vi "MP_SYNCHRONISED_TEST.vi"(5 "error in (no error)":errorcluster, 6 "TB: IP ADDRESS":string="192.168.0.100", 7 "Chopper Serial Number":string="26", 8 "Connection ID TB":refnum<k5>, 9 "Connection ID CC":refnum<k5>) -> (0 "PASS / FAIL":bool, 1 "error out":errorcluster, 2 "Connection ID CC 2":refnum<k5>, 3 "Connection ID TB 2":refnum<k5>, 4 "concatenated string":string)   [LabVIEW 2013]
panel:
  out "PROGRESS":i32(slide) scale=0.0..5.0
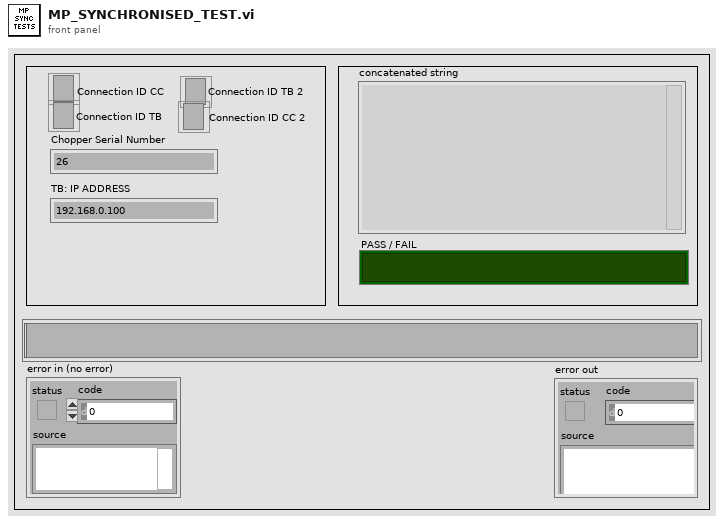
[diagram p1: front panel]
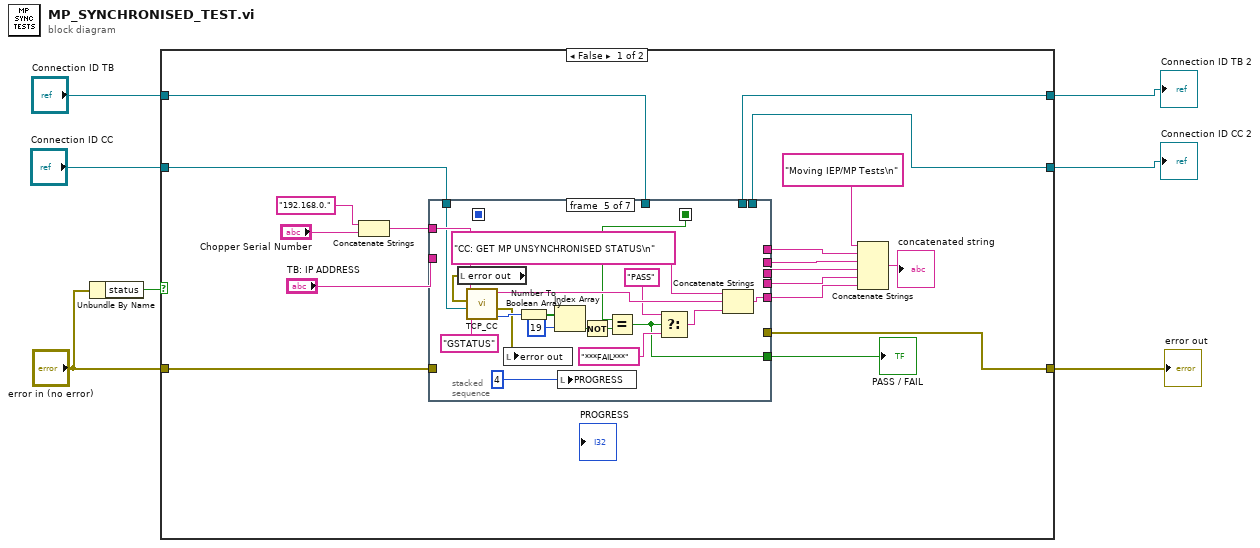
[diagram p0: block diagram]
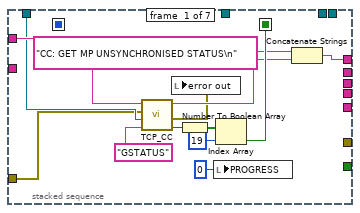
[diagram p2: hidden frame]
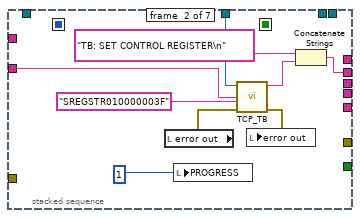
[diagram p3: hidden frame]
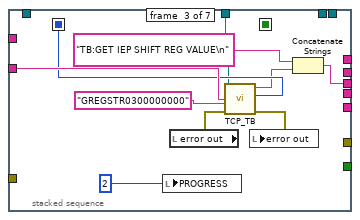
[diagram p4: hidden frame]
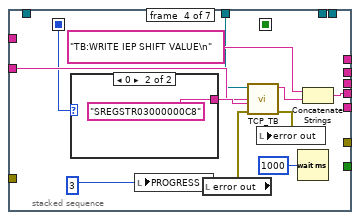
[diagram p5: hidden frame]
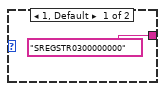
[diagram p6: hidden frame]
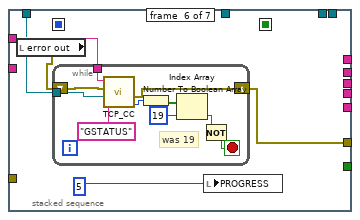
[diagram p7: hidden frame]
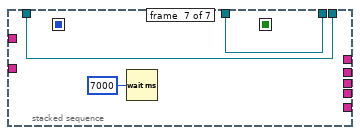
[diagram p8: hidden frame]
diagram:
  n1 = Unbundle By Name("error in (no error)") -> ("status"=w2:bool)
  n2 = case shown="False" w2 {
    tunnel: "Connection ID CC" -> [w13 w109]
    tunnel: "Connection ID TB" -> [w12 w110]
    tunnel: [w9 w110] -> w5
    tunnel: [w8 w109] -> w4
    tunnel: "error in (no error)" -> [w11 w108]
    tunnel: [w10 w108] -> w3
    frame False {
      n3 = Concatenate Strings("192.168.0.", "Chopper Serial Number") -> (w14:string)
      n4 = stacked-sequence {
        seq-local: [w33 _ _ _ _ _ _] -> [_ _ _ _ w79 _ _]
        seq-local: [_ _ w55 _ _ _ _] -> [_ _ _ w66 _ _ _]
        tunnel: "TB: IP ADDRESS" -> [_ w46 w56 w67 _ _ _]
        tunnel: w14 -> [w37 _ _ _ w88 w94 _]
        tunnel: [w30 _ _ _ _ _ _] -> w25
        tunnel: [_ w43 _ _ _ _ _] -> w24
        tunnel: [_ _ w52 _ _ _ _] -> w23
        tunnel: [_ _ _ w63 _ _ _] -> w22
        tunnel: [_ _ _ _ w82 _ _] -> w21
        tunnel: [_ _ _ _ w75 _ _] -> w16
        tunnel: w13 -> [w28 _ _ _ w73 w92 w105]
        tunnel: w12 -> [_ w41 w50 w60 _ _ w106]
        tunnel: w11 -> [w27 _ _ _ _ _ _]
        tunnel: [_ _ _ _ _ w91 _] -> w10
        tunnel: [_ _ _ _ _ _ w106] -> w9
        tunnel: [_ _ _ _ _ _ w105] -> w8
        frame #0 {
          n5 = call "TCP_CC.vi"("COMMAND"="GSTATUS", "connection ID"=w28, "error in (no error)"=w27, "IP ADDRESS"=w37) -> ("number"=w36:u32, "error out"=w26:errorcluster, "The Response:"=w31:string)  [unwired: 1 out]
          n6 = local write "error out"(w26) -> ()
          n7 = Number To Boolean Array(number=w36) -> (Boolean array=w35:bool[])
          n8 = local write "PROGRESS"(0 ("PROGRESS")) -> ()
          n9 = Index Array(array=w35, index=19) -> (element=w33:bool)
          n10 = Concatenate Strings("CC: GET MP UNSYNCHRONISED STATUS\n", w31) -> (w30:string)
        }
        frame #1 {
          n11 = local read "error out"() -> (w39:errorcluster)
          n12 = local write "PROGRESS"(1 ("PROGRESS")) -> ()
          n13 = call "TCP_TB.vi"("IP ADDRESS"=w46, "error in (no error)"=w39, "COMMAND"="SREGSTR010000003F", "Connection ID IN"=w41) -> ("error out"=w40:errorcluster, "Their Response:"=w44:string)  [unwired: 2 in, 1 out]
          n14 = local write "error out"(w40) -> ()
          n15 = Concatenate Strings("TB: SET CONTROL REGISTER\n" ("COMMAND"), w44) -> (w43:string)
        }
        frame #2 {
          n16 = local write "PROGRESS"(2 ("PROGRESS")) -> ()
          n17 = local read "error out"() -> (w48:errorcluster)
          n18 = call "TCP_TB.vi"("IP ADDRESS"=w56, "error in (no error)"=w48, "COMMAND"="GREGSTR0300000000", "Connection ID IN"=w50) -> ("error out"=w49:errorcluster, "Decimal Number"=w55:u32, "Their Response:"=w54:string)  [unwired: 2 in]
          n19 = local write "error out"(w49) -> ()
          n20 = Concatenate Strings("TB:GET IEP SHIFT REG VALUE\n" ("COMMAND"), w54) -> (w52:string)
        }
        frame #3 {
          n21 = case shown="0" w66 {
            tunnel: ["SREGSTR0300000000" ("COMMAND") "SREGSTR03000000C8" ("COMMAND")] -> w68
            frame 1, Default {
            }
            frame 0 {
            }
          }
          n22 = local write "PROGRESS"(3 ("PROGRESS")) -> ()
          n23 = local read "error out"() -> (w58:errorcluster)
          n24 = call "TCP_TB.vi"("IP ADDRESS"=w67, "error in (no error)"=w58, "COMMAND"=w68, "Connection ID IN"=w60) -> ("error out"=w59:errorcluster, "Their Response:"=w65:string)  [unwired: 2 in, 1 out]
          n25 = local write "error out"(w59) -> ()
          n26 = Wait (ms)(milliseconds to wait=u32 1000 ("millisecond multiple")) -> ()  [unwired: 1 out]
          n27 = Concatenate Strings("TB:WRITE IEP SHIFT VALUE\n", w65) -> (w63:string)
        }
        frame #4 {
          n28 = local read "error out"() -> (w71:errorcluster)
          n29 = call "TCP_CC.vi"("COMMAND"="GSTATUS", "connection ID"=w73, "error in (no error)"=w71, "IP ADDRESS"=w88) -> ("number"=w87:u32, "error out"=w72:errorcluster, "The Response:"=w83:string)  [unwired: 1 out]
          n30 = local write "error out"(w72) -> ()
          n31 = Number To Boolean Array(number=w87) -> (Boolean array=w86:bool[])
          n32 = Index Array(array=w86, index=19) -> (element=w81:bool)
          n33 = local write "PROGRESS"(4 ("PROGRESS")) -> ()
          n34 = Not(x=w81) -> (.not. x?=w80:bool)
          n35 = Equal?(x=w79, y=w80) -> (x = y?=w75:bool)
          n36 = Select(t="PASS", s=w75, f="***FAIL***") -> (s? t:f=w76:string)
          n37 = Concatenate Strings("CC: GET MP UNSYNCHRONISED STATUS\n", w83, w76) -> (w82:string)
        }
        frame #5 {
          n38 = local read "error out"() -> (w90:errorcluster)
          n39 = while {
            tunnel: w94 -> [w100]
            tunnel: w92 -> [w97]
            shift-right: [w96] -> w91
            shift-left: w90 -> [w95]
            stop <- w98 stop-if-true
            # "was 19"
            n40 = call "TCP_CC.vi"("COMMAND"="GSTATUS", "connection ID"=w97, "error in (no error)"=w95, "IP ADDRESS"=w100) -> ("number"=w103:u32, "error out"=w96:errorcluster)  [unwired: 2 out]
            n41 = Number To Boolean Array(number=w103) -> (Boolean array=w102:bool[])
            n42 = Index Array(array=w102, index=19) -> (element=w99:bool)
            n43 = Not(x=w99) -> (.not. x?=w98:bool)
          }
          n44 = local write "PROGRESS"(5 ("PROGRESS")) -> ()
        }
        frame #6 {
          n45 = Wait (ms)(milliseconds to wait=u32 7000 ("millisecond multiple")) -> ()  [unwired: 1 out]
        }
      }
      "PASS / FAIL" <- w16
      n46 = Concatenate Strings("Moving IEP/MP Tests\n", w25, w24, w23, w22, w21) -> (→"concatenated string":string)
    }
    frame True {
    }
  }
  "Connection ID TB 2" <- w5
  "Connection ID CC 2" <- w4
  "error out" <- w3
